vi "watch dog.vi"   [LabVIEW 2018]
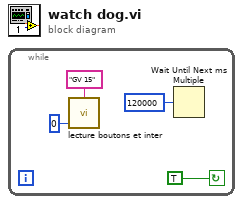
[diagram p0: block diagram]
diagram:
  n1 = while {
    stop <- TRUE continue-if-true
    n2 = call "lecture boutons et inter.vi"("com #"=0, "Entrée Commande"="GV 15") -> ()  [unwired: 1 in, 1 out]
    n3 = Wait Until Next ms Multiple(millisecond multiple=u32 120000 ("n millisecondes")) -> ()  [unwired: 1 out]
  }
